vi "test_DmmInstrument_CallInitializeMeasurementLinkSessionWithCreateBehavior_RemoteSessionCreated.vi"(8 "error in":errorcluster) -> (0 "error out":errorcluster, 2 "result":string, 3 "pass":bool)   [LabVIEW 2020, in "MeasurementServerTests.lvlib"]
uses:
  MeasurementServerTests.lvlib
  Runtime/Sessions/niDMM Sessions/Session Factory/Session Factory.lvclass
  Runtime/Sessions/Instrument Sessions/ISession Factory/Initialize and Close Session Behavior.ctl
  Runtime/Sessions/Instrument Sessions/ISession Factory/ISession Factory.lvclass
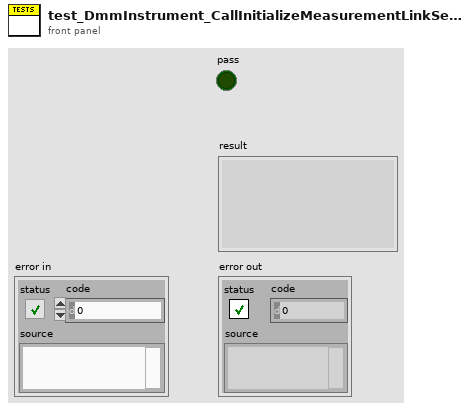
[diagram p1: front panel]
types:
  T1 = typedef "Plug-In SDK Instrument Sessions.lvlib/ISession Factory.lvclass/Remote Connection Options.ctl" = cluster{"session name":string, "address":string, "port":u32}
  T2 = typedef "Plug-In SDK Instrument Sessions.lvlib/ISession Factory.lvclass/Initialize and Close Session Behavior.ctl" = enum16{"Initialize and Close", "Attach and Detach", "Initialize and Detach", "Attach and Close"}
  T3 = typedef "Plug-In SDK Instrument Sessions.lvlib/ISession Factory.lvclass/Session Initialization Parameters.ctl" = cluster{"resource name":string, "session name":string}
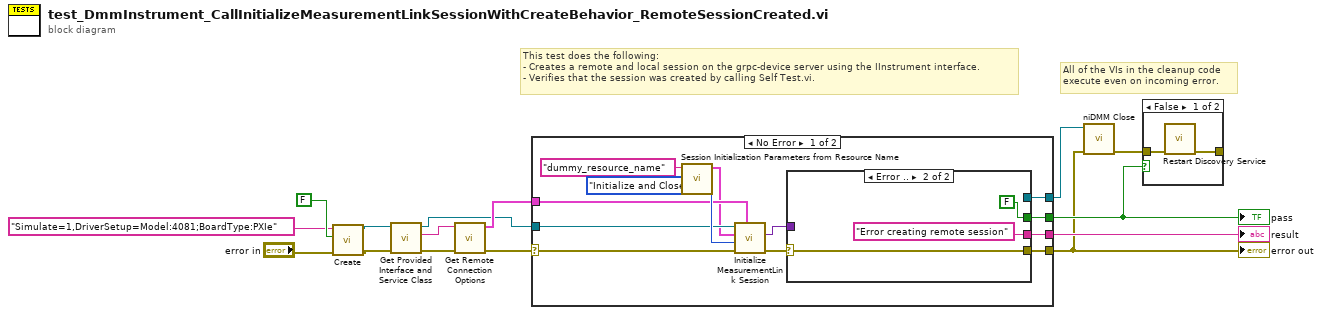
[diagram p0: block diagram]
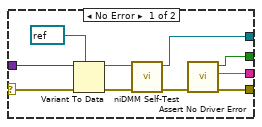
[diagram p2: hidden frame]
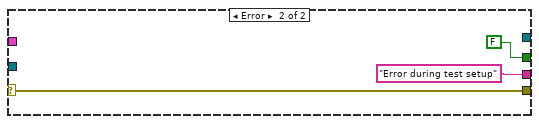
[diagram p3: hidden frame]
diagram:
  # "All of the VIs in the cleanup code\nexecute even on incoming error."
  # "This test does the following:\n- Creates a remote and local session on the grpc-device server using the IInstrument interface.\n- Verifies that the session was created by calling Self Test.vi."
  n1 = call "Create.vi"("error in"="error in", "reset"=FALSE, "option string"="Simulate=1,DriverSetup=Model:4081;BoardType:PXIe") -> ("error out"=w5:errorcluster, "session factory out"=w6:refnum<class "Session Factory.lvclass">)  [unwired: 7 in]
  n2 = call-dynamic "Get Provided Interface and Service Class.vi"("error in"=w5, "session factory in"=w6) -> ("error out"=w13:errorcluster, "provided interface"=w14:string, "session factory out"=w10:refnum<class "Session Factory.lvclass">)  [unwired: 6 in, 1 out]
  n3 = call "Get Remote Connection Options.vi"("error in"=w13, "provided interface"=w14) -> ("error out"=w12:errorcluster, "remote connection options"=w11:T1)  [unwired: 8 in]
  n4 = case shown="No Error" w12 {
    selector: w12 -> [w20 w41]
    tunnel: [w26 w41] -> w7
    tunnel: [w27 FALSE] -> w8
    tunnel: [w25 "Error during test setup" ("f")] -> w15
    tunnel: w11 -> [w19 _]
    tunnel: w10 -> [w18 _]
    tunnel: [w17 _] -> w1
    frame No Error {
      n5 = call "Session Initialization Parameters from Resource Name.vi"("resource name"="dummy_resource_name") -> ("session initialization parameters"=w16:T3)  [unwired: 10 in]
      n6 = call-dynamic "Initialize MeasurementLink Session.vi"("remote connection options"=w19, "error in"=w20, "initialize and close session behavior"=Initialize_and_Close_Session_Behavior."Initialize and Close", "session initialization parameters"=w16, "session factory in"=w18) -> ("error out"=w23:errorcluster, "session out"=w24:variant)  [unwired: 4 in, 1 out]
      n7 = case shown="Error .." w23 {
        selector: w23 -> [w34 w39]
        tunnel: [w37 FALSE] -> w27
        tunnel: [w32 w39] -> w26
        tunnel: [w36 "Error creating remote session"] -> w25
        tunnel: w24 -> [w35 _]
        tunnel: [w31 _] -> w17
        frame No Error {
          n8 = Variant To Data(error in=w34, type=refnum<k15> refnum, Variant=w35) -> (data=w29:refnum<k15>, error out=w33:errorcluster)
          n9 = call <instrlib>:"niDMM Self-Test.vi"("error in (no error)"=w33, "instrument handle"=w29) -> ("error out"=w30:errorcluster, "instrument handle out"=w31:refnum<k15>)  [unwired: 6 in, 2 out]
          n10 = call "Assert No Driver Error.vi"("error in"=w30) -> ("error out"=w32:errorcluster, "result"=w36:string, "pass?"=w37:bool)  [unwired: 8 in]
        }
        frame Error {
        }
      }
    }
    frame Error {
    }
  }
  "error out" <- w7
  "pass" <- w8
  "result" <- w15
  n11 = call <instrlib>:"niDMM Close.vi"("error in (no error)"=w7, "instrument handle"=w1) -> ("error out"=w9:errorcluster)  [unwired: 9 in]
  n12 = case shown="False" w8 {
    tunnel: w9 -> [w45 _]
    tunnel: [w44 _] -> _
    frame False {
      n13 = call "Restart Discovery Service.vi"("error in"=w45) -> ("error out"=w44:errorcluster)  [unwired: 10 in]
    }
    frame True {
    }
  }
